vi "tx_dac_couping.vi"(1 "Enum":enum16{"B2A", "A2B"}(ring), 2 "fs":dbl=125000000.0, 3 "error in (no error)":errorcluster caption="错误输入（无错误）", 4 "fin":dbl[](array[numeric])=[218000000.0, 215000000.0, 220000000.0, 225000000.0, 230000000.0, 235000000.0, 240000000.0, 205000000.0, 200000000.0], 5 "开关":bool[](array[boolean])=[FALSE, TRUE, TRUE, FALSE, FALSE, FALSE, FALSE, TRUE, TRUE, FALSE], 6 "VISA resource name 2":refnum<visa-resource-name>="COM3" caption="VISA资源名称") -> (0 "error out":errorcluster={"status"=FALSE, "code"=1047, "source"=""})   [LabVIEW 2015]
uses:
  <vilib>/Instr/_visa.llb/VISA Configure Serial Port (Instr).vi
panel:
  out "连接的字符串":string
  out "VI":dbl[](array[numeric])
  out "Real":dbl
  out "CFG_RAM":bool
  out "TXPLL_INIT":bool
  out "DLL_MAN":bool
  out "EXT_CLK":bool
  in  "选项卡控件":enum32{"选项卡 1", "选项卡 2"}(tab)
  out "RF_out":dbl[](array[numeric])
  out "HQ":dbl[](array[numeric])
  out "HI":dbl[](array[numeric])
  out "VQ":dbl[](array[numeric])
  out "num_of_samples":dbl
  out "two":dbl
  out "predist":dbl
  out "one":dbl=1.0
  out "ten":dbl
  out "four":dbl
  out "three":dbl
  out "VISA resource name out":refnum<visa-resource-name>="COM3"
  # "EXT_CLK"
  # "TXPLL_INIT"
  # "ONE_TONE"
  # "TWO_TONE"
  # "THREE_TONE"
  # "FOUR_TONE"
  # "TEN_TONE"
  # "CFG_RAM"
  # "DLL_MAN"
  # "PREDIST"
  # "external clk&dll manul"
  # "external clk&dll auto"
  # "internal clk&dll manual"
  # "internal clk&dll auto"
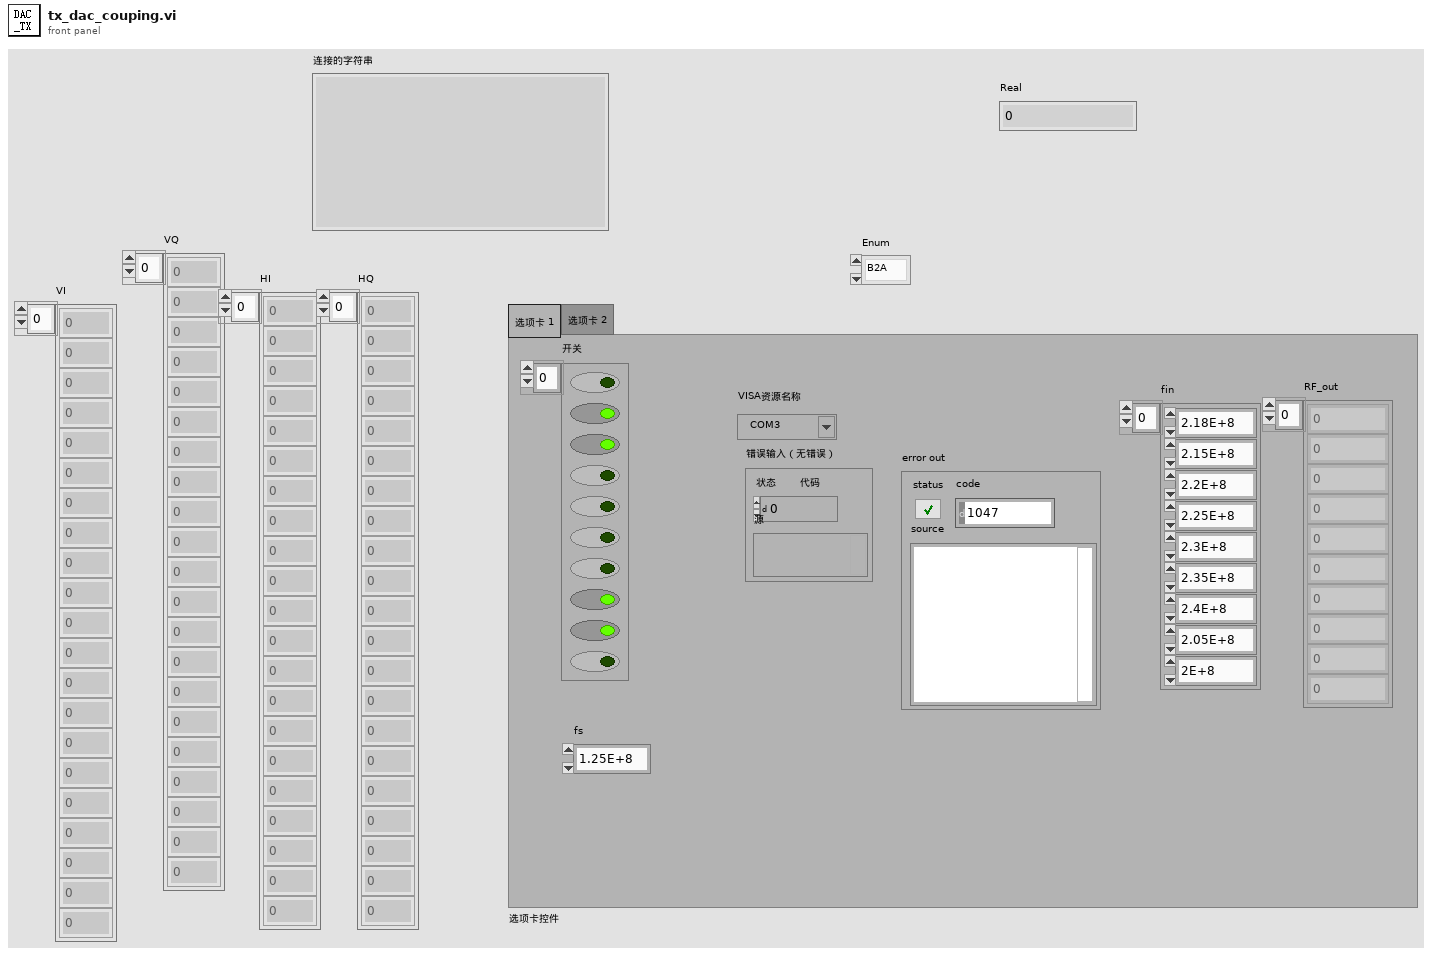
[diagram p1: front panel]
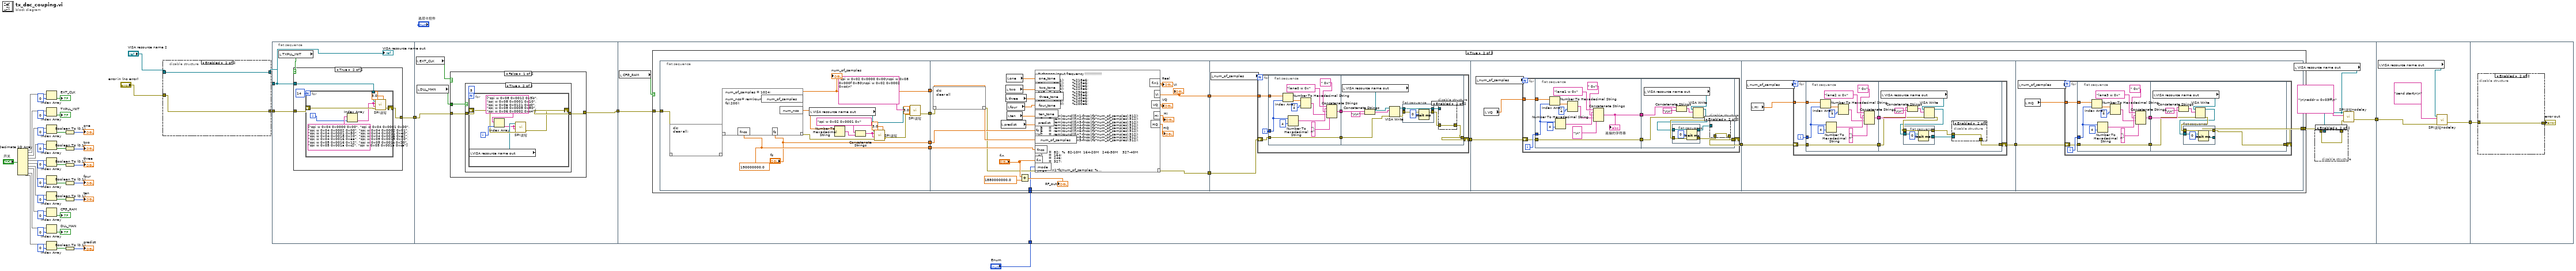
[diagram p0: block diagram]
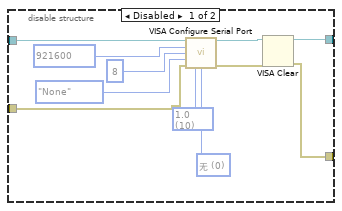
[diagram p2: hidden frame]
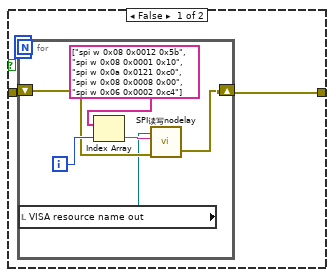
[diagram p4: hidden frame]
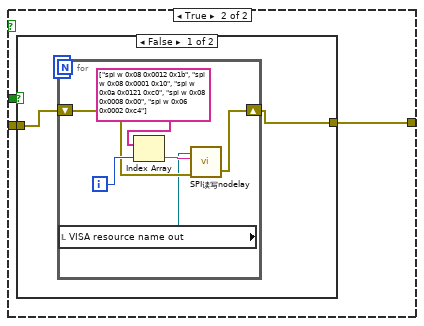
[diagram p5: hidden frame]
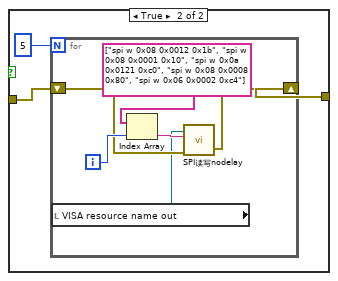
[diagram p6: hidden frame]
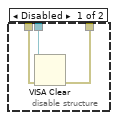
[diagram p7: hidden frame]
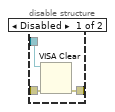
[diagram p9: hidden frame]
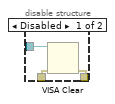
[diagram p10: hidden frame]
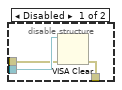
[diagram p11: hidden frame]
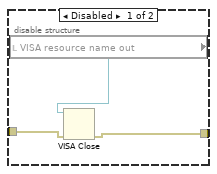
[diagram p12: hidden frame]
diagram:
  n1 = Decimate 1D Array("开关") -> (w33:bool[], w29:bool[], w26:bool[], w25:bool[], w23:bool[], w21:bool[], w19:bool[], w16:bool[], w13:bool[], w11:bool[])
  n2 = Index Array(array=w33, index=0 ("索引")) -> (element=→"EXT_CLK":bool)
  n3 = Index Array(array=w29, index=0 ("索引")) -> (element=→"TXPLL_INIT":bool)
  n4 = Index Array(array=w26, index=0 ("索引")) -> (element=w9:bool)
  n5 = Index Array(array=w25, index=0 ("索引")) -> (element=w8:bool)
  n6 = Index Array(array=w23, index=0 ("索引")) -> (element=w7:bool)
  n7 = Index Array(array=w21, index=0 ("索引")) -> (element=w6:bool)
  n8 = Index Array(array=w19, index=0 ("索引")) -> (element=w5:bool)
  n9 = Index Array(array=w16, index=0 ("索引")) -> (element=→"CFG_RAM":bool)
  n10 = Index Array(array=w13, index=0 ("索引")) -> (element=→"DLL_MAN":bool)
  n11 = Index Array(array=w11, index=0 ("索引")) -> (element=w4:bool)
  n12 = Boolean To (0,1)(Boolean=w9) -> (0, 1=→"one":i16)
  n13 = Boolean To (0,1)(Boolean=w8) -> (0, 1=→"two":i16)
  n14 = Boolean To (0,1)(Boolean=w7) -> (0, 1=→"three":i16)
  n15 = Boolean To (0,1)(Boolean=w6) -> (0, 1=→"four":i16)
  n16 = Boolean To (0,1)(Boolean=w5) -> (0, 1=→"ten":i16)
  n17 = Boolean To (0,1)(Boolean=w4) -> (0, 1=→"predist":i16)
  n18 = disable-structure shown="Enabled" {
    disable-tunnel: "VISA resource name 2" -> [w50 w59]
    disable-tunnel: "error in (no error)" -> [w49 w58]
    disable-tunnel: [w48 w59] -> w44
    disable-tunnel: [w47 w58] -> w43
    frame Disabled {
      w53 = u16 0 items=["无", "XON/XOFF", "RTS/CTS", "XON/XOFF & RTS/CTS", "DTR/DSR", "XON/XOFF & DTR/DSR"] ("flow control (0:none)")
      w54 = u16 10 items=["1.0"=10, "1.5"=15, "2.0"=20] ("stop bits (10: 1 bit)")
      n19 = call-poly "VISA Configure Serial Port"("VISA resource name"=w50, "baud rate (9600)"=u32 921600, "data bits (8)"=u16 8, "parity (0:none)"=enum16{"None", "Odd", "Even", "Mark", "Space"}."None", "error in (no error)"=w49, "stop bits (10: 1 bit)"=w54, "flow control (0:none)"=w53) -> ("VISA resource name out"=w52:refnum<visa-resource-name>, "error out"=w51:errorcluster)  [unwired: 7 in]
      n20 = VISA Clear(VISA resource name=w52, error in (no error)=w51) -> (VISA resource name out=w48:refnum<visa-resource-name>, error out=w47:errorcluster)
    }
    frame Enabled {
    }
  }
  n21 = flat-sequence {
    tunnel: w44 -> [w60]
    tunnel: w43 -> [w63]
    tunnel: [w62] -> w42
    tunnel: w42 -> [w79]
    tunnel: [w76] -> w3
    tunnel: [w127] -> w35
    tunnel: w3 -> [w129]
    tunnel: "Enum" -> [w122]
    tunnel: w35 -> [w335]
    tunnel: [w334] -> w2
    tunnel: w2 -> [w339]
    frame #0 {
      n22 = local read "TXPLL_INIT"() -> (w61:bool)
      n23 = case shown="True" w61 {
        tunnel: w60 -> [_ w68]
        tunnel: w63 -> [w64 w67]
        tunnel: [w64 w66] -> w62
        frame False {
        }
        frame True {
          n24 = for {
            N: 14 -> [_]
            tunnel: w68 -> [w70]
            shift-right: [w73] -> w66
            shift-left: w67 -> [w72]
            i -> [w74]
            n25 = Index Array(array=string[] ["spi w 0x04 0x0000 0x00", "spi w 0x04 0x0001 0x00", "spi w 0x04 0x0002 0x00", "spi w 0x04 0x0002 0x01", "spi w 0x04 0x0001 0x80", "spi w 0x04 0x0011 0xe0", "spi w 0x04 0x0018 0x20", "spi w 0x04 0x0016 0xe2", "spi w 0x04 0x0016 0xea", "spi w 0x05 0x0015 0x20", "spi w 0x05 0x0016 0x12", "spi w 0x05 0x001c 0x20", "spi w 0x05 0x001a 0xc2", "spi w 0x05 0x001a 0xca"], index=w74) -> (element=w71:string)
            n26 = call "SPI读写.vi"("DELAY"=3.0, "error in (no error)"=w72, "从芯片读数据"=w71, "往芯片写数据"=w71, "VISA resource name"=w70) -> ("error out"=w73:errorcluster)  [unwired: 1 out]
          }
        }
      }
      "VISA resource name out" <- w60
    }
    frame #1 {
      n27 = local read "EXT_CLK"() -> (w78:bool)
      n28 = local read "DLL_MAN"() -> (w77:bool)
      n29 = case shown="False" w78 {
        tunnel: w77 -> [w82 w103]
        tunnel: [w81 w102] -> w76
        tunnel: w79 -> [w80 w101]
        frame False {
          n30 = case shown="True" w82 {
            tunnel: [w84 w92] -> w81
            tunnel: w80 -> [w85 w93]
            frame False {
              n31 = for {
                N: 5 -> [_]
                shift-right: [w87] -> w84
                shift-left: w85 -> [w88]
                i -> [w91]
                n32 = local read "VISA resource name out"() -> (w86:refnum<visa-resource-name>)
                n33 = Index Array(array=string[] ["spi w 0x08 0x0012 0x5b", "spi w 0x08 0x0001 0x10", "spi w 0x0a 0x0121 0xc0", "spi w 0x08 0x0008 0x00", "spi w 0x06 0x0002 0xc4"], index=w91) -> (element=w89:string)
                n34 = call "SPI读写nodelay.vi"("error in (no error)"=w88, "往芯片写数据"=w89, "VISA resource name"=w86) -> ("error out"=w87:errorcluster)  [unwired: 1 in, 1 out]
              }
            }
            frame True {
              n35 = for {
                N: 5 -> [_]
                shift-right: [w98] -> w92
                shift-left: w93 -> [w97]
                i -> [w100]
                n36 = local read "VISA resource name out"() -> (w96:refnum<visa-resource-name>)
                n37 = Index Array(array=string[] ["spi w 0x08 0x0012 0x5b", "spi w 0x08 0x0001 0x10", "spi w 0x0a 0x0121 0xc0", "spi w 0x08 0x0008 0x80", "spi w 0x06 0x0002 0xc4"], index=w100) -> (element=w95:string)
                n38 = call "SPI读写.vi"("error in (no error)"=w97, "从芯片读数据"=w95, "往芯片写数据"=w95, "VISA resource name"=w96) -> ("error out"=w98:errorcluster)  [unwired: 1 in, 1 out]
              }
            }
          }
        }
        frame True {
          n39 = case shown="False" w103 {
            tunnel: [w105 w114] -> w102
            tunnel: w101 -> [w106 w115]
            frame False {
              n40 = for {
                N: 5 -> [_]
                shift-right: [w108] -> w105
                shift-left: w106 -> [w109]
                i -> [w112]
                n41 = local read "VISA resource name out"() -> (w107:refnum<visa-resource-name>)
                n42 = Index Array(array=string[] ["spi w 0x08 0x0012 0x1b", "spi w 0x08 0x0001 0x10", "spi w 0x0a 0x0121 0xc0", "spi w 0x08 0x0008 0x00", "spi w 0x06 0x0002 0xc4"], index=w112) -> (element=w110:string)
                n43 = call "SPI读写nodelay.vi"("error in (no error)"=w109, "往芯片写数据"=w110, "VISA resource name"=w107) -> ("error out"=w108:errorcluster)  [unwired: 1 in, 1 out]
              }
            }
            frame True {
              n44 = for {
                N: 5 -> [_]
                shift-right: [w117] -> w114
                shift-left: w115 -> [w118]
                i -> [w121]
                n45 = local read "VISA resource name out"() -> (w116:refnum<visa-resource-name>)
                n46 = Index Array(array=string[] ["spi w 0x08 0x0012 0x1b", "spi w 0x08 0x0001 0x10", "spi w 0x0a 0x0121 0xc0", "spi w 0x08 0x0008 0x80", "spi w 0x06 0x0002 0xc4"], index=w121) -> (element=w119:string)
                n47 = call "SPI读写nodelay.vi"("error in (no error)"=w118, "往芯片写数据"=w119, "VISA resource name"=w116) -> ("error out"=w117:errorcluster)  [unwired: 1 in, 1 out]
              }
            }
          }
        }
      }
    }
    frame #2 {
      n48 = local read "CFG_RAM"() -> (w126:bool)
      n49 = case shown="True" w126 {
        tunnel: w129 -> [w134 w146]
        tunnel: [w134 w141] -> w124
        tunnel: w122 -> [_ w135]
        frame False {
        }
        frame True {
          n50 = flat-sequence {
            tunnel: w146 -> [w157]
            tunnel: [w154] -> w145
            tunnel: [w159] -> w144
            tunnel: ["fs"] -> w137
            tunnel: [w158] -> w136
            tunnel: w145 -> [w165]
            tunnel: w144 -> [w183]
            tunnel: [w176] -> w143
            tunnel: [w175] -> w142
            tunnel: w137 -> [w171]
            tunnel: w136 -> [w170]
            tunnel: w135 -> [w163]
            tunnel: w143 -> [w185]
            tunnel: w142 -> [w186]
            tunnel: [w184] -> w138
            tunnel: [w224] -> w139
            tunnel: w138 -> [w223]
            tunnel: [w263] -> w140
            tunnel: w139 -> [w262]
            tunnel: [w302] -> w141
            tunnel: w140 -> [w301]
            frame #0 {
              w158 = 190000000.0 ("fnco")
              w153 = "spi w 0x02 0x0000 0x00\nspi w 0x08 0x000f 0x80\nspi w 0x02 0x0002 0xcc\n" ("往芯片写数据")
              n51 = script code="clc;\nclear all;"("??"=w157) -> ("??"=w156:errorcluster)
              n52 = script code="num_of_samples = 1024;\n\nnum_nco= rem(round(fnco/5e6*125e6/fs),200);"("??"=w156, "fnco"=w158, "fs"="fs") -> ("??"=w148:errorcluster, "num_of_samples"=w159:dbl, "num_nco"=w160:dbl)
              "num_of_samples" <- w159
              n53 = local read "VISA resource name out"() -> (w150:refnum<visa-resource-name>)
              n54 = Number To Hexadecimal String(2:w160) -> (0:w162:string)  [unwired: 1 in]
              n55 = Concatenate Strings("spi w 0x02 0x0001 0x", w162) -> (w151:string)
              n56 = call "SPI读写.vi"("DELAY"=3.0, "error in (no error)"=w148, "从芯片读数据"=w151, "往芯片写数据"=w151, "VISA resource name"=w150) -> ("error out"=w149:errorcluster)  [unwired: 1 out]
              n57 = call "SPI读写.vi"("DELAY"=3.0, "error in (no error)"=w149, "从芯片读数据"=w153, "往芯片写数据"=w153, "VISA resource name"=w150) -> ("error out"=w154:errorcluster)  [unwired: 1 out]
            }
            frame #1 {
              n58 = script code="clc;\nclear all"("??"=w165) -> ("??"=w164:errorcluster)
              n59 = local read "predist"() -> (w177:dbl)
              n60 = local read "three"() -> (w180:dbl)
              n61 = local read "two"() -> (w181:dbl)
              n62 = local read "one"() -> (w182:dbl)
              n63 = local read "four"() -> (w179:dbl)
              n64 = local read "ten"() -> (w178:dbl)
              n65 = Add(x="fin", y=1880000000.0) -> (x+y=→"RF_out":dbl[])
              n66 = script code="%change input frequency!!!!!!!!!!!!!!!\n\nfin1   =  fin(1);       %218e6;\nfin2   =  fin(2);       %215e6;\nfin3   =  fin(3);       %220e6;\nfin4   =  fin(4);       %225e6;\nfin5   =  fin(5);       %230e6;\nfin6   =  fin(6);       %235e6;\nfin7   =  fin(7);       %240e6;\nfin8   =  fin(8);       %205e6;\nfin9   =  fin(9);       %200e6;\n\n\n\nn1     =  rem(round((fin1-fnco)/fs*num_of_samples),512);\nn2     =  rem(round((fin2-fnco)/fs*num_of_samples),512);\nn3     =  rem(round((fin3-fnco)/fs*num_of_samples),512);\nn4     =  rem(round((fin4-fnco)/fs*num_of_samples),512);\nn5     =  rem(round((fin5-fnco)/fs*num_of_samples),512);\nn6     =  rem(round((fin6-fnco)/fs*num_of_samples),512);\nn7     =  rem(round((fin7-fnco)/fs*num_of_samples),512);\nn8     =  rem(round((fin8-fnco)/fs*num_of_samples),512);\nn9     =  rem(round((fin9-fnco)/fs*num_of_samples),512);\n\n\nif 0\nn1     =  82;  %  82-10M  164-20M   246-30M    327-40M\nn2     =  164;\nn3     =  246;\nn4     =  327;\nend\n\nfsig1 = n1*fs/num_of_samples; % \nfsig2 = n2*fs/num_of_samples;  % \nfsig3 = n3*fs/num_of_samples;\nfsig4 = n4*fs/num_of_samples;\nfsig5 = n5*fs/num_of_samples;\nfsig6 = n6*fs/num_of_samples;\nfsig7 = n7*fs/num_of_samples;\nfsig8 = n8*fs/num_of_samples;\nfsig9 = n9*fs/num_of_samples;\n\n\n\nbits = 14;\namp  = -1;\n\n\nif one_tone\n    amp = -1;   %%% dBFs default:-1\nend\nif two_tone\n    amp = -10.2;   %%% dBFs default:-1\nend\nif three_tone\n    amp = -9.2;   %%% dBFs default:-1\nend\nif four_tone\n    amp = -16;   %%% dBFs default:-1\nend\n\nf1 = (0:1:num_of_samples-1)*fsig1/fs*2*pi;\nf2 = (0:1:num_of_samples-1)*fsig2/fs*2*pi;\nf3 = (0:1:num_of_samples-1)*fsig3/fs*2*pi;\nf4 = (0:1:num_of_samples-1)*fsig4/fs*2*pi;\nf5 = (0:1:num_of_samples-1)*fsig5/fs*2*pi;\nf6 = (0:1:num_of_samples-1)*fsig6/fs*2*pi;\nf7 = (0:1:num_of_samples-1)*fsig7/fs*2*pi;\nf8 = (0:1:num_of_samples-1)*fsig8/fs*2*pi;\nf9 = (0:1:num_of_samples-1)*fsig9/fs*2*pi;\n\nf1_dly = ((0:1:num_of_samples-1)+0.74)*fsig1/fs*2*pi;\nf2_dly = ((0:1:num_of_samples-1)+0.59)*fsig2/fs*2*pi;\nf3_dly = ((0:1:num_of_samples-1)+0.74)*fsig3/fs*2*pi;\nf4_dly = ((0:1:num_of_samples-1)+0.59)*fsig4/fs*2*pi;\n\n\n\namp_dig = round(2^(bits-1)*10^(amp/20));\namp_dig2 = round(2^(bits-1)*10^((amp-0)/20));\namp_dig3 = round(2^(bits-1)*10^((amp-0)/20));\namp_dig4 = round(2^(bits-1)*10^((amp-0)/20));\n\n\n if(one_tone)\n     LHP_I = round(amp_dig*(cos(f1)));\n     LHP_Q = round(amp_dig*(cos(f1)));\n     RHP_I = round(amp_dig*(sin(f1)));\n     RHP_Q = round(amp_dig*(sin(f1)));\n     \n     \n          \n elseif(two_tone)\n     LHP_I = round(amp_dig*(cos(f1))+amp_dig2*(cos(f2)));\n     LHP_Q = round(amp_dig*(cos(f1))+amp_dig2*(cos(f2)));\n     RHP_I = round(amp_dig*(sin(f1))+amp_dig2*(sin(f2)));\n     RHP_Q = round(amp_dig*(sin(f1))+amp_dig2*(sin(f2)));\n \n     \n     \n elseif(three_tone)\n     LHP_I = round(amp_dig*(cos(f1))+amp_dig2*(cos(f2))+amp_dig3*(cos(f3)));\n     LHP_Q = round(amp_dig*(sin(f2))+amp_dig2*(cos(f2))+amp_dig3*(cos(f3)));\n     RHP_I = round(amp_dig*(sin(f3))+amp_dig2*(sin(f2))+amp_dig3*(sin(f3)));\n     RHP_Q = round(amp_dig*(sin(f4))+amp_dig2*(sin(f2))+amp_dig3*(sin(f3)));\n     \n elseif(four_tone)\n     LHP_I = round(amp_dig*(cos(f1))+amp_dig2*(cos(f2))+amp_dig3*(cos(f3))+amp_dig4*(cos(f4)));\n     LHP_Q = round(amp_dig*(cos(f1))+amp_dig2*(cos(f2))+amp_dig3*(cos(f3))+amp_dig4*(cos(f4)));\n     RHP_I = round(amp_dig*(sin(f1))+amp_dig2*(sin(f2))+amp_dig3*(sin(f3))+amp_dig4*(sin(f4)));\n     RHP_Q = round(amp_dig*(sin(f1))+amp_dig2*(sin(f2))+amp_dig3*(sin(f3))+amp_dig4*(sin(f4)));\n  \n         \n elseif(ten_tone)  \n      LHP_I = round(amp_dig*(cos(f1))+amp_dig2*(cos(f2))+amp_dig3*(cos(f3))+amp_dig4*(cos(f4))+amp_dig4*(cos(f5))+amp_dig4*(cos(f6))+amp_dig4*(cos(f7))+amp_dig4*(cos(f8))+amp_dig4*(cos(f9)));\n      LHP_Q = round(amp_dig*(cos(f1))+amp_dig2*(cos(f2))+amp_dig3*(cos(f3))+amp_dig4*(cos(f4))+amp_dig4*(cos(f5))+amp_dig4*(cos(f6))+amp_dig4*(cos(f7))+amp_dig4*(cos(f8))+amp_dig4*(cos(f9)));\n      RHP_I = round(amp_dig*(cos(f1))+amp_dig2*(cos(f2))+amp_dig3*(cos(f3))+amp_dig4*(cos(f4))+amp_dig4*(cos(f5))+amp_dig4*(cos(f6))+amp_dig4*(cos(f7))+amp_dig4*(cos(f8))+amp_dig4*(cos(f9)));\n      RHP_Q = round(amp_dig*(cos(f1))+amp_dig2*(cos(f2))+amp_dig3*(cos(f3))+amp_dig4*(cos(f4))+amp_dig4*(cos(f5))+amp_dig4*(cos(f6))+amp_dig4*(cos(f7))+amp_dig4*(cos(f8))+amp_dig4*(cos(f9)));\n     \n\n else\n     LHP_I = round(amp_dig*(cos(f1)));\n     LHP_Q = round(amp_dig*(cos(f2)));\n     RHP_I = round(amp_dig*(sin(f3)));\n     RHP_Q = round(amp_dig*(sin(f4)));\n\n end\n \n  VI = (LHP_I + RHP_I)/2; \n  VQ = (RHP_Q - LHP_Q)/2;\n  HI = (LHP_I + RHP_I)/2; \n  HQ = (RHP_Q - LHP_Q)/2;\n  \n  if(predist)\n      k_final1 = -19.58;\n      k_final2 = -19.98;   \n      amp_final1 = round(2^(bits-1)*10^(k_final1/20));\n      amp_final2 = round(2^(bits-1)*10^(k_final2/20));  \n  \n      if(two_tone)\n          LHP_I_dly = round(amp_dig*(cos(f1_dly))+amp_dig2*(cos(f2_dly)));\n          LHP_Q_dly = round(amp_dig*(cos(f1_dly))+amp_dig2*(cos(f2_dly)));\n          RHP_I_dly = round(amp_dig*(sin(f1_dly))+amp_dig2*(sin(f2_dly)));\n          RHP_Q_dly = round(amp_dig*(sin(f1_dly))+amp_dig2*(sin(f2_dly)));    \n      elseif(four_tone)\n          LHP_I_dly = round(amp_dig*(cos(f1_dly))+amp_dig2*(cos(f2_dly))+amp_dig3*(cos(f3_dly))+amp_dig4*(cos(f4_dly)));\n          LHP_Q_dly = round(amp_dig*(cos(f1_dly))+amp_dig2*(cos(f2_dly))+amp_dig3*(cos(f3_dly))+amp_dig4*(cos(f4_dly)));\n          RHP_I_dly = round(amp_dig*(sin(f1_dly))+amp_dig2*(sin(f2_dly))+amp_dig3*(sin(f3_dly))+amp_dig4*(sin(f4_dly)));\n          RHP_Q_dly = round(amp_dig*(sin(f1_dly))+amp_dig2*(sin(f2_dly))+amp_dig3*(sin(f3_dly))+amp_dig4*(sin(f4_dly)));  \n      end\n  \n      VI_dly = (LHP_I_dly + RHP_I_dly)/2; \n      VQ_dly = (RHP_Q_dly - LHP_Q_dly)/2;\n      HI_dly = (LHP_I_dly + RHP_I_dly)/2; \n      HQ_dly = (RHP_Q_dly - LHP_Q_dly)/2;  \n   \n      VI = VI + round(amp_final1*(VI_dly/8192).^3) ;\n      VQ = VQ + round(amp_final2*(VQ_dly/8192).^3) ;\n      HI = HI + round(amp_final1*(HI_dly/8192).^3);\n      HQ = HQ + round(amp_final2*(HQ_dly/8192).^3) ;\n  end\n    \nif mode == 1\n  VI = 0*round(VI); \n  VQ =0* round(VQ); \nelse\n  HI =0* round(HI); \n  HQ =0* round(HQ); \nend\n  \n  VI(find(VI<0))=VI(find(VI<0))+16384;\n  VQ(find(VQ<0))=VQ(find(VQ<0))+16384;\n  HI(find(HI<0))=HI(find(HI<0))+16384;\n  HQ(find(HQ<0))=HQ(find(HQ<0))+16384;"("??"=w164, "one_tone"=w182, "two_tone"=w181, "three_tone"=w180, "four_tone"=w179, "ten_tone"=w178, "predist"=w177, "fs"=w171, "num_of_samples"=w183, "fnco"=w170, "fin"="fin", "mode"=w163) -> ("??"=w176:errorcluster, "VI"=w175:dbl[], "VQ"=→"VQ":dbl[], "HI"=→"HI":dbl[], "HQ"=→"HQ":dbl[], "fin1"=→"Real":dbl)
              "VI" <- w175
            }
            frame #2 {
              n67 = local read "num_of_samples"() -> (w187:dbl)
              n68 = for {
                N: w187 -> [_]
                tunnel: w186 -> [w192]
                shift-right: [w188] -> w184
                shift-left: w185 -> [w189]
                i -> [w193]
                n69 = flat-sequence {
                  tunnel: w193 -> [w204]
                  tunnel: w192 -> [w203]
                  tunnel: [w195] -> w191
                  tunnel: [w194] -> w190
                  tunnel: w189 -> [w194]
                  tunnel: w191 -> [w214]
                  tunnel: w190 -> [w211]
                  tunnel: [w206] -> w188
                  frame #0 {
                    n70 = Index Array(array=w203, index=w204) -> (element=w201:dbl)
                    n71 = Number To Hexadecimal String(1:i16 4 ("宽度(-)"), 2:w204) -> (0:w200:string)
                    n72 = Number To Hexadecimal String(1:i16 4 ("宽度(-)"), 2:w201) -> (0:w198:string)
                    n73 = Concatenate Strings("lane0 w 0x" ("字符串"), w200, " 0x" ("字符串"), w198, "\n" ("字符串")) -> (w195:string)
                  }
                  frame #1 {
                    n74 = local read "VISA resource name out"() -> (w215:refnum<visa-resource-name>)
                    n75 = Concatenate Strings(w214, "\r\n") -> (w212:string)
                    n76 = VISA Write(VISA resource name=w215, write buffer=w212, error in (no error)=w211) -> (VISA resource name out=w210:refnum<visa-resource-name>, error out=w209:errorcluster)  [unwired: 1 out]
                    n77 = flat-sequence {
                      tunnel: [w221] -> w208
                      tunnel: w210 -> [w221]
                      tunnel: [w220] -> w207
                      tunnel: w209 -> [w220]
                      frame #0 {
                        n78 = Wait (ms)(milliseconds to wait=u32 0 ("等待时间（毫秒）")) -> ()  [unwired: 1 out]
                      }
                    }
                    n79 = disable-structure shown="Enabled" {
                      disable-tunnel: w208 -> [w218 _]
                      disable-tunnel: w207 -> [w217 w219]
                      disable-tunnel: [w216 w219] -> w206
                      frame Disabled {
                        n80 = VISA Clear(VISA resource name=w218, error in (no error)=w217) -> (error out=w216:errorcluster)  [unwired: 1 out]
                      }
                      frame Enabled {
                      }
                    }
                  }
                }
              }
            }
            frame #3 {
              n81 = local read "num_of_samples"() -> (w226:dbl)
              n82 = local read "VQ"() -> (w225:dbl[])
              n83 = for {
                N: w226 -> [_]
                tunnel: w225 -> [w231]
                shift-right: [w227] -> w224
                shift-left: w223 -> [w228]
                i -> [w232]
                n84 = flat-sequence {
                  tunnel: w232 -> [w243]
                  tunnel: w231 -> [w242]
                  tunnel: [w234] -> w230
                  tunnel: [w233] -> w229
                  tunnel: w228 -> [w233]
                  tunnel: w230 -> [w254]
                  tunnel: w229 -> [w250]
                  tunnel: [w245] -> w227
                  frame #0 {
                    n85 = Index Array(array=w242, index=w243) -> (element=w240:dbl)
                    n86 = Number To Hexadecimal String(1:i16 4 ("宽度(-)"), 2:w243) -> (0:w239:string)
                    n87 = Number To Hexadecimal String(1:i16 4 ("宽度(-)"), 2:w240) -> (0:w237:string)
                    n88 = Concatenate Strings("lane1 w 0x" ("字符串"), w239, " 0x" ("字符串"), w237, "\n" ("字符串")) -> (w234:string)
                    "连接的字符串" <- w234
                  }
                  frame #1 {
                    n89 = local read "VISA resource name out"() -> (w251:refnum<visa-resource-name>)
                    n90 = flat-sequence {
                      tunnel: [w260] -> w246
                      tunnel: w249 -> [w260]
                      tunnel: [w259] -> w247
                      tunnel: w248 -> [w259]
                      frame #0 {
                        n91 = Wait (ms)(milliseconds to wait=u32 0 ("等待时间（毫秒）")) -> ()  [unwired: 1 out]
                      }
                    }
                    n92 = Concatenate Strings(w254, "\r\n") -> (w252:string)
                    n93 = VISA Write(VISA resource name=w251, write buffer=w252, error in (no error)=w250) -> (VISA resource name out=w248:refnum<visa-resource-name>, error out=w249:errorcluster)  [unwired: 1 out]
                    n94 = disable-structure shown="Enabled" {
                      disable-tunnel: w247 -> [w257 _]
                      disable-tunnel: w246 -> [w256 w258]
                      disable-tunnel: [w255 w258] -> w245
                      frame Disabled {
                        n95 = VISA Clear(VISA resource name=w257, error in (no error)=w256) -> (error out=w255:errorcluster)  [unwired: 1 out]
                      }
                      frame Enabled {
                      }
                    }
                  }
                }
              }
            }
            frame #4 {
              n96 = local read "num_of_samples"() -> (w265:dbl)
              n97 = local read "HI"() -> (w264:dbl[])
              n98 = for {
                N: w265 -> [_]
                tunnel: w264 -> [w270]
                shift-right: [w266] -> w263
                shift-left: w262 -> [w267]
                i -> [w271]
                n99 = flat-sequence {
                  tunnel: w271 -> [w282]
                  tunnel: w270 -> [w281]
                  tunnel: [w273] -> w269
                  tunnel: [w272] -> w268
                  tunnel: w267 -> [w272]
                  tunnel: w269 -> [w291]
                  tunnel: w268 -> [w290]
                  tunnel: [w284] -> w266
                  frame #0 {
                    n100 = Index Array(array=w281, index=w282) -> (element=w279:dbl)
                    n101 = Number To Hexadecimal String(1:i16 4 ("宽度(-)"), 2:w282) -> (0:w278:string)
                    n102 = Number To Hexadecimal String(1:i16 4 ("宽度(-)"), 2:w279) -> (0:w276:string)
                    n103 = Concatenate Strings("lane2 w 0x" ("字符串"), w278, " 0x" ("字符串"), w276, "\n" ("字符串")) -> (w273:string)
                  }
                  frame #1 {
                    n104 = local read "VISA resource name out"() -> (w289:refnum<visa-resource-name>)
                    n105 = flat-sequence {
                      tunnel: [w299] -> w285
                      tunnel: w288 -> [w299]
                      tunnel: [w298] -> w286
                      tunnel: w287 -> [w298]
                      frame #0 {
                        n106 = Wait (ms)(milliseconds to wait=u32 0 ("等待时间（毫秒）")) -> ()  [unwired: 1 out]
                      }
                    }
                    n107 = Concatenate Strings(w291, "\r\n") -> (w293:string)
                    n108 = VISA Write(VISA resource name=w289, write buffer=w293, error in (no error)=w290) -> (VISA resource name out=w287:refnum<visa-resource-name>, error out=w288:errorcluster)  [unwired: 1 out]
                    n109 = disable-structure shown="Enabled" {
                      disable-tunnel: w286 -> [w296 _]
                      disable-tunnel: w285 -> [w295 w297]
                      disable-tunnel: [w294 w297] -> w284
                      frame Disabled {
                        n110 = VISA Clear(VISA resource name=w296, error in (no error)=w295) -> (error out=w294:errorcluster)  [unwired: 1 out]
                      }
                      frame Enabled {
                      }
                    }
                  }
                }
              }
            }
            frame #5 {
              n111 = local read "num_of_samples"() -> (w304:dbl)
              n112 = local read "HQ"() -> (w303:dbl[])
              n113 = for {
                N: w304 -> [_]
                tunnel: w303 -> [w309]
                shift-right: [w305] -> w302
                shift-left: w301 -> [w306]
                i -> [w310]
                n114 = flat-sequence {
                  tunnel: w310 -> [w321]
                  tunnel: w309 -> [w320]
                  tunnel: [w312] -> w308
                  tunnel: [w311] -> w307
                  tunnel: w306 -> [w311]
                  tunnel: w308 -> [w328]
                  tunnel: w307 -> [w326]
                  tunnel: [w323] -> w305
                  frame #0 {
                    n115 = Index Array(array=w320, index=w321) -> (element=w318:dbl)
                    n116 = Number To Hexadecimal String(1:i16 4 ("宽度(-)"), 2:w321) -> (0:w317:string)
                    n117 = Number To Hexadecimal String(1:i16 4 ("宽度(-)"), 2:w318) -> (0:w315:string)
                    n118 = Concatenate Strings("lane3 w 0x" ("字符串"), w317, " 0x" ("字符串"), w315, "\n" ("字符串")) -> (w312:string)
                  }
                  frame #1 {
                    n119 = local read "VISA resource name out"() -> (w327:refnum<visa-resource-name>)
                    n120 = Concatenate Strings(w328, "\r\n") -> (w329:string)
                    n121 = flat-sequence {
                      tunnel: [w332] -> w323
                      tunnel: w325 -> [w332]
                      tunnel: [w331] -> _
                      tunnel: w324 -> [w331]
                      frame #0 {
                        n122 = Wait (ms)(milliseconds to wait=u32 0 ("等待时间（毫秒）")) -> ()  [unwired: 1 out]
                      }
                    }
                    n123 = VISA Write(VISA resource name=w327, write buffer=w329, error in (no error)=w326) -> (VISA resource name out=w324:refnum<visa-resource-name>, error out=w325:errorcluster)  [unwired: 1 out]
                  }
                }
              }
            }
          }
        }
      }
      n124 = local read "VISA resource name out"() -> (w123:refnum<visa-resource-name>)
      n125 = disable-structure shown="Enabled" {
        disable-tunnel: [w132 w133] -> w125
        disable-tunnel: w124 -> [w131 w133]
        disable-tunnel: w123 -> [w130 _]
        frame Disabled {
          n126 = VISA Clear(VISA resource name=w130, error in (no error)=w131) -> (error out=w132:errorcluster)  [unwired: 1 out]
        }
        frame Enabled {
        }
      }
      n127 = call "SPI读写nodelay.vi"("error in (no error)"=w125, "往芯片写数据"="\n\naddr w 0x03ff\n", "VISA resource name"=w123) -> ("error out"=w127:errorcluster)  [unwired: 1 in, 1 out]
    }
    frame #3 {
      n128 = local read "VISA resource name out"() -> (w336:refnum<visa-resource-name>)
      n129 = call "SPI读写nodelay.vi"("error in (no error)"=w335, "往芯片写数据"="send start\n\n", "VISA resource name"=w336) -> ("error out"=w334:errorcluster)  [unwired: 1 in, 1 out]
    }
    frame #4 {
      n130 = disable-structure shown="Enabled" {
        disable-tunnel: w339 -> [w342 w343]
        disable-tunnel: [w341 w343] -> w338
        frame Disabled {
          n131 = local read "VISA resource name out"() -> (w340:refnum<visa-resource-name>)
          n132 = VISA Close(VISA resource name=w340, error in (no error)=w342) -> (error out=w341:errorcluster)
        }
        frame Enabled {
        }
      }
      "error out" <- w338
    }
  }
